vi "Register Discovery Events.vi"(8 "error in (no error)":errorcluster, 11 "CIFPluginManager in":refnum<class "CIFPluginManager.lvclass">) -> (0 "error out":errorcluster, 2 "Event Registration Refnum":refnum<event-registration>, 3 "CIFPluginManager out":refnum<class "CIFPluginManager.lvclass">)   [LabVIEW 2021, in "CIFPluginManager.lvclass"]
uses:
  CIFPluginManager.lvclass
  typedef/Discover Command.ctl
  CIFPluginManager.lvclass/CIFPluginManager.ctl
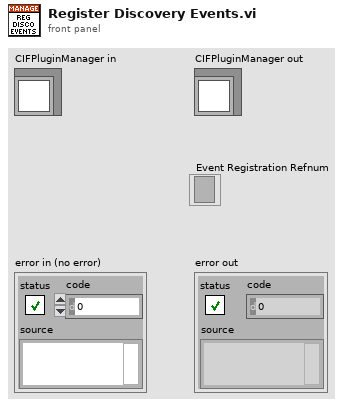
[diagram p1: front panel]
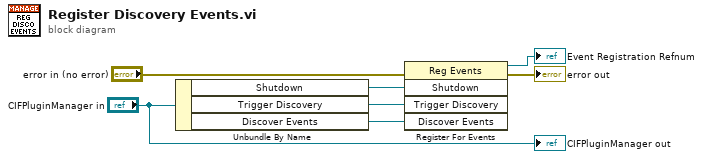
[diagram p0: block diagram]
diagram:
  n1 = Unbundle By Name("CIFPluginManager in") -> ("Shutdown"=w4:refnum<user-event>, "Trigger Discovery"=w7:refnum<user-event>, "Discover Events"=w2:refnum<user-event>)
  n2 = register-events(error in="error in (no error)", w4, w7, w2) -> (reference out=→"Event Registration Refnum":refnum<event-registration>, error out=→"error out":errorcluster)  [unwired: 1 in]
  "CIFPluginManager out" <- "CIFPluginManager in"
